vi "Calibrate Adc Data Query.vi"(8 "error in":errorcluster, 10 "Interleave":i32 caption="Interleave Method", 11 "Instrument Handle In":i32) -> (0 "error out":errorcluster, 1 "Q Gain Code":u16, 2 "I Gain Code":u16, 3 "Instrument Handle Out":i32, 4 "Q Zero Code":u16, 5 "I Zero Code":u16)   [LabVIEW 8.6, in "ZTScopeM.lvlib"]
doc: "Query the instrument's ADC calibration codes. See the instrument calibration manual for more information."
uses:
  ZTScopeM.lvlib
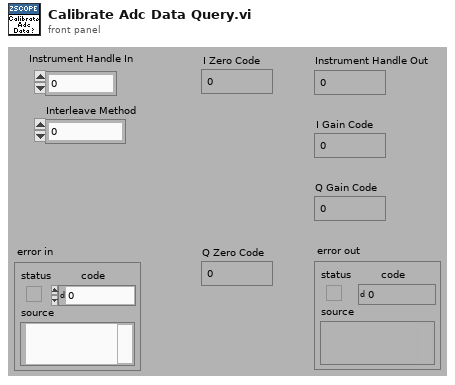
[diagram p1: front panel]
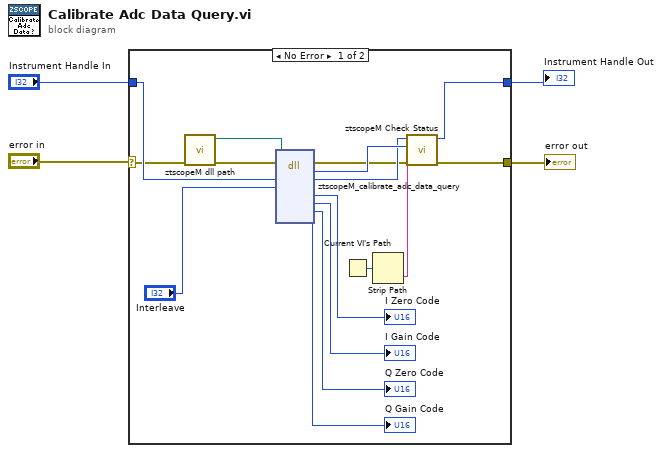
[diagram p0: block diagram]
diagram:
  n1 = case shown="No Error" "error in" {
    selector: "error in" -> [w8 w22]
    tunnel: [w15 w22] -> w1
    tunnel: "Instrument Handle In" -> [w20 w21]
    tunnel: [w14 w21] -> w3
    frame #0 {
      n2 = call "ztscopeM dll path.vi"("error in (no error)"=w8) -> ("error out"=w6:errorcluster, "<instrument>.dll path"=w7:path)  [unwired: 9 in]
      n3 = dll-call lib="C:/Program Files (x86)/National Instruments/LabVIEW 2013/instr.lib/ztscopem/ztscopeM.dll" fn="ztscopeM_calibrate_adc_data_query"(path in=w7, error in=w6, "instrumentHandle"=w20, "Interleave Method"="Interleave") -> (error out=w5:errorcluster, w17:i32, "instrumentHandle"=w16:i32, "I Zero Code"=→"I Zero Code":u16, "I Gain Code"=→"I Gain Code":u16, "Q Zero Code"=→"Q Zero Code":u16, "Q Gain Code"=→"Q Gain Code":u16)  [unwired: 6 in, 1 out]
      n4 = Current VI's Path() -> (path=w19:path)
      n5 = Strip Path(path=w19) -> (name=w18:string)  [unwired: 1 out]
      n6 = call "ztscopeM Check Status.vi"("error in"=w5, "name of VI"=w18, "status (return code)"=w17, "instrument handle in"=w16) -> ("error out"=w15:errorcluster, "instrument handle out"=w14:i32)  [unwired: 2 in]
    }
    frame #1 {
    }
  }
  "Instrument Handle Out" <- w3
  "error out" <- w1
